vi "RT PWM Host.vi"() -> ()   [LabVIEW 2025]
uses:
  FPGA IP/Types/PWM.Generate.Digital.Convert.Settings.ctl
  FPGA IP/Types/PWM.Measure.Digital.Result.ctl
  <vilib>/FPGAPlugInAG/cRIO-9045/niLvFpga_Open_cRIO-9045.vi
  <vilib>/rvi/interface/common/dynamic/niFpgaDynamicAddResources.vi
  <vilib>/Utility/error.llb/Error Cluster From Error Code.vi
  <vilib>/rvi/errors/niLvFpgaAdjustHostInterfaceError.vi
  <vilib>/FPGAPlugInAG/Dynamic/niLvFpga_Close_Dynamic.vi
  <vilib>/rvi/interface/nirviOpenFPGA/nirviOpenFPGA.xnode
  FPGA Bitfiles/pwmsexamplecode_FPGATarget_FPGAPWMs_Q1V+ZO8nIss.lvbitx
  FPGA PWMs.vi
  <vilib>/rvi/interface/nirviReadWriteControl/nirviReadWriteControl.xnode
  <vilib>/rvi/interface/nirviCloseFPGA/nirviCloseFPGA.xnode
  <vilib>/rvi/interface/Simulation/niFpgaSimulationCallBeginRW.vi
  FPGA IP/Speciality FPGA IO.lvlib
  NiFpgaLv.dll
panel:
  out "Mod2 DI3 PWM Measurement":T1
  out "Mod2 DI0 PWM Measurement":T1
  in  "Mod2 PWM Gen Settings":T2={"ACTIVE EDGE"=TRUE, "FREQ"=10000.0, "DC"=25.0}
  in  "Mod1 PWM Gen Settings":T2={"ACTIVE EDGE"=TRUE, "FREQ"=500.0, "DC"=50.0}
  out "error out":errorcluster
  in  "stop":bool
  in  "Mod2 DI3 PWM AcqSettings":cluster{"ACTIVE EDGE":bool, "TIMEOUT":u32}={"ACTIVE EDGE"=TRUE, "TIMEOUT"=40000000}
  in  "Mod2 DI0 PWM AcqSettings":cluster{"ACTIVE EDGE":bool, "TIMEOUT":u32}={"ACTIVE EDGE"=TRUE, "TIMEOUT"=40000000}
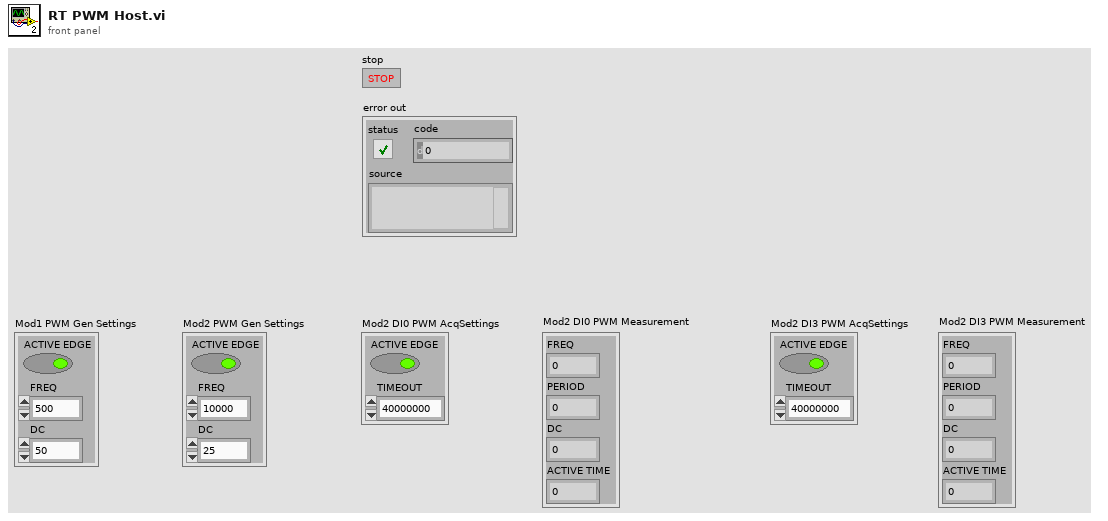
[diagram p1: front panel]
types:
  T1 = typedef "Speciality FPGA IO.lvlib/PWM.Measure.Digital.Result.ctl" = cluster{"FREQ":sgl, "PERIOD":sgl, "DC":sgl, "ACTIVE TIME":sgl}
  T2 = typedef "Speciality FPGA IO.lvlib/PWM.Generate.Digital.Convert.Settings.ctl" = cluster{"ACTIVE EDGE":bool, "FREQ":sgl, "DC":sgl}
  T3 = typedef "Speciality FPGA IO.lvlib/PWM.Generate.Digital.Settings.ctl" = cluster{"ACTIVE EDGE":bool, "ACTIVE TICKS":u32, "INACTIVE TICKS":u32}
  T4 = cluster{"ACTIVE TICKS":u32, "INACTIVE TICKS":u32, "ACQ TICKS":u32}
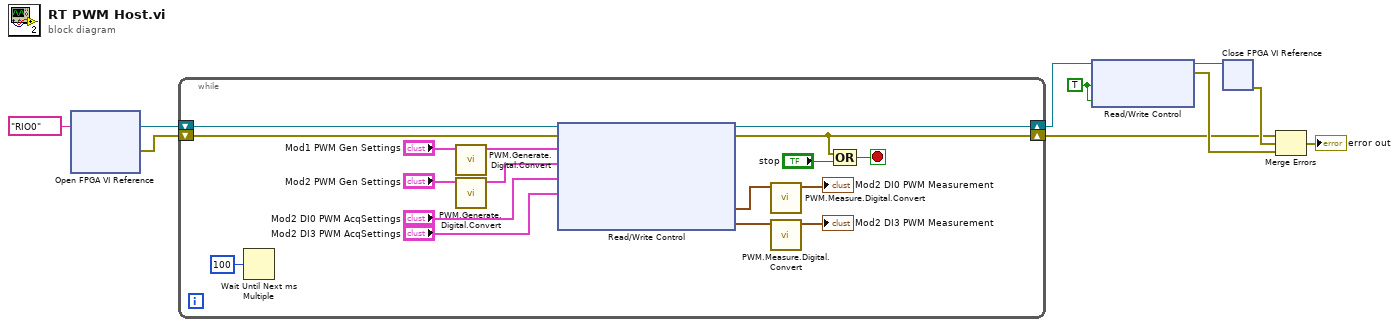
[diagram p0: block diagram]
diagram:
  w6 = TRUE ("Stop Slow PWM")
  n1 = xnode "Open FPGA VI Reference"("resource name"=tag "RIO0") -> ("FPGA VI Reference Out"=w9:refnum<k20>, "error out"=w8:errorcluster)  [unwired: 1 in]
  n2 = while {
    shift-right: [w25] -> w7
    shift-left: w9 -> [w27]
    shift-right: [w21] -> w2
    shift-left: w8 -> [w26]
    stop <- w19 stop-if-true
    n3 = Wait Until Next ms Multiple(millisecond multiple=u32 100) -> ()  [unwired: 1 out]
    n4 = call "PWM.Generate.Digital.Convert.vi"("Settings"="Mod1 PWM Gen Settings") -> ("Settings"=w18:T3)  [unwired: 10 in]
    n5 = call "PWM.Generate.Digital.Convert.vi"("Settings"="Mod2 PWM Gen Settings") -> ("Settings"=w16:T3)  [unwired: 10 in]
    n6 = xnode "Read/Write Control"("FPGA VI Reference In"=w27, "error in"=w26, "Mod1 PWM Gen Settings"=w18, "Mod2 PWM Gen Settings"=w16, "Mod2 DI0 PWM AcqSettings"="Mod2 DI0 PWM AcqSettings", "Mod2 DI3 PWM AcqSettings"="Mod2 DI3 PWM AcqSettings") -> ("FPGA VI Reference Out"=w25:refnum<k20>, "error out"=w21:errorcluster, "Mod2 DI0 PWM Measurement"=w14:T4, "Mod2 DI3 PWM Measurement"=w13:T4)
    n7 = call "PWM.Measure.Digital.Convert.vi"("Measurement"=w14) -> ("Result"=→"Mod2 DI0 PWM Measurement":T1)  [unwired: 10 in]
    n8 = call "PWM.Measure.Digital.Convert.vi"("Measurement"=w13) -> ("Result"=→"Mod2 DI3 PWM Measurement":T1)  [unwired: 10 in]
    n9 = Compound Arithmetic op=OR(w21, "stop") -> (w19:bool)
  }
  n10 = xnode "Read/Write Control"("FPGA VI Reference In"=w7, "Stop Slow PWM"=w6, "Stop Fast PWM"=w6) -> ("FPGA VI Reference Out"=w5:refnum<k20>, "error out"=w3:errorcluster)  [unwired: 1 in]
  n11 = xnode "Close FPGA VI Reference"("FPGA VI Reference In"=w5) -> ("error out"=w4:errorcluster)  [unwired: 1 in]
  n12 = Merge Errors(w2, w4, w3) -> (→"error out":errorcluster)
